vi "report_generierung.vi"(1 "Not-Aus betätigt":dbl, 2 "fehlbearbeitungen":i32, 3 "bearbeitung gestartedt":dbl, 4 "start zeit":timestamp) -> (0 "String":string)   [LabVIEW 2010]
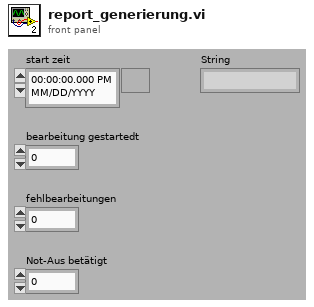
[diagram p1: front panel]
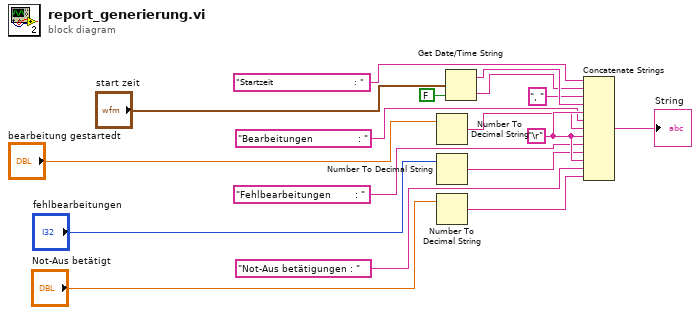
[diagram p0: block diagram]
diagram:
  w15 = "\r"
  n1 = Number To Decimal String(number="bearbeitung gestartedt") -> (decimal integer string=w9:string)  [unwired: 1 out]
  n2 = Number To Decimal String(number="fehlbearbeitungen") -> (decimal integer string=w14:string)  [unwired: 1 out]
  n3 = Number To Decimal String(number="Not-Aus betätigt") -> (decimal integer string=w17:string)  [unwired: 1 out]
  n4 = Get Date/Time String(seconds (now)="start zeit", want seconds? (F)=FALSE ("Angabe von Sekunden? (F)")) -> (date string=w8:string, time string=w5:string)  [unwired: 1 out]
  n5 = Concatenate Strings("Startzeit                           : " ("String"), w5, ", " ("String"), w8, w15, "Bearbeitungen               : " ("String"), w9, w15, "Fehlbearbeitungen        : " ("String"), w14, w15, "Not-Aus betätigungen : " ("String"), w17) -> (→"String":string)
